vi "Host Key Hash.vi"(8 "Error In":errorcluster, 10 "Type":T1=enum."SHA1", 11 "Session In":refnum<class "Session.lvclass">) -> (0 "Error Out":errorcluster, 2 "Hash":u8[](array[numeric]) format="%.0x", 3 "Sesssion Out":refnum<class "Session.lvclass">)   [LabVIEW 2017, in "LabSSH2.lvlib" / "Session.lvclass"]
uses:
  Session.lvclass
  Typedefs/Host Key Hash Types.ctl
  Session.lvclass/Session.ctl
  <vilib>/Utility/error.llb/Error Cluster From Error Code.vi
  <vilib>/ErrorRing/Error Ring.xnode
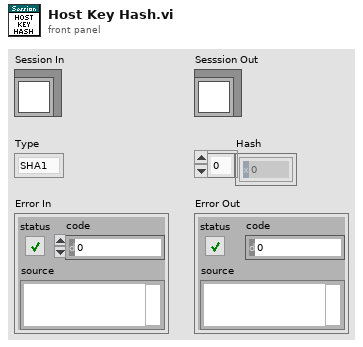
[diagram p1: front panel]
types:
  T1 = typedef "LabSSH2.lvlib/Session.lvclass/Host Key Hash Types.ctl" = enum16{"MD5", "SHA1"}
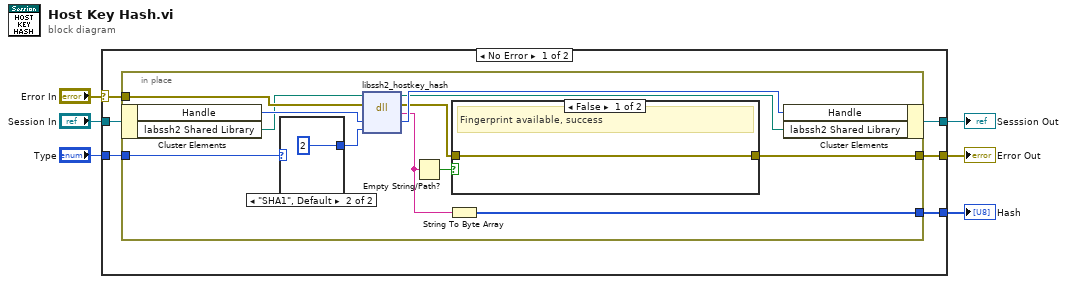
[diagram p0: block diagram]
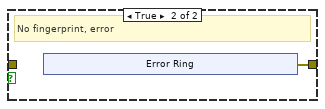
[diagram p2: hidden frame]
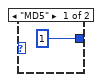
[diagram p3: hidden frame]
diagram:
  n1 = case shown="No Error" "Error In" {
    selector: "Error In" -> [w11 w34]
    tunnel: [w12 w34] -> w5
    tunnel: "Session In" -> [w10 w33]
    tunnel: [w9 w33] -> w3
    tunnel: "Type" -> [w8 _]
    tunnel: [w7 _] -> w1
    frame No Error {
      n2 = in-place {
        in-place-border: [w15] -> w12
        in-place-border: w11 -> [w24]
        in-place-border: w8 -> [w19]
        in-place-border: [w13] -> w7
        n3 = in-place-cluster #1(w10) -> ("Handle"=w23:u64, "labssh2 Shared Library"=w21:path)
        n4 = case shown="\"SHA1\", Default" w19 {
          tunnel: [1 2] -> w18
          frame "MD5" {
          }
          frame "SHA1", Default {
          }
        }
        n5 = dll-call lib="D:/Users/cfield/Code/Field R&D Services/SSH/LabSSH2/LabVIEW/trunk/src/LabSSH2/Private/labssh2.*" fn="libssh2_hostkey_hash"(path in=w21, error in=w24, "session"=w23, "hash_type"=w18) -> (path out=w20:path, error out=w16:errorcluster, "fingerprint"=w14:string, "session"=w22:u64)  [unwired: 2 in]
        n6 = Empty String/Path?(string/path=w14) -> (empty?=w17:bool)
        n7 = String To Byte Array(string=w14) -> (unsigned byte array=w13:u8[])
        n8 = case shown="False" w17 {
          tunnel: w16 -> [w25 _]
          tunnel: [w25 w26] -> w15
          frame False {
            # "Fingerprint available, success"
          }
          frame True {
            # "No fingerprint, error"
            n9 = xnode "Error Ring"() -> ("error out"=w26:errorcluster)
          }
        }
        n10 = in-place-cluster #1("Handle"=w22, "labssh2 Shared Library"=w20) -> (w9:refnum<class "Session.lvclass">)
      }
    }
    frame Error {
    }
  }
  "Sesssion Out" <- w3
  "Error Out" <- w5
  "Hash" <- w1
